vi "Update Call Chain.vi"(8 "error in (no error)":errorcluster, 11 "Data Cluster in":T1={"PeekVI Reference"=refnum, "SubPanel"=refnum, "Peek Stack Tree Ref"=refnum, "Open Button Ref"=refnum, "Top VI"=refnum, "Active VI"=refnum, "Stack"=[], "Last FP State"=enum."Standard"}) -> (0 "error out":errorcluster, 3 "Data Cluster out":T1={"PeekVI Reference"=refnum, "SubPanel"=refnum, "Peek Stack Tree Ref"=refnum, "Open Button Ref"=refnum, "Top VI"=refnum, "Active VI"=refnum, "Stack"=[], "Last FP State"=enum."Standard"})   [LabVIEW 2020, in "Peek Window.lvlib"]
uses:
  Peek Window.lvlib
  MHL Data Cluster.ctl
  VI Types/Standard VI Type/Standard VI Type.lvclass
  <vilib>/Utility/traverseref.llb/TRef TravTarget.ctl
  VI Types/Standard VI Type/Standard VI Type.lvclass/Standard VI Type.ctl
  VI Types/Standard VI Type/Read Full Qualified Name.vi
  <vilib>/Utility/traverseref.llb/VI Scripting - Traverse.lvlib
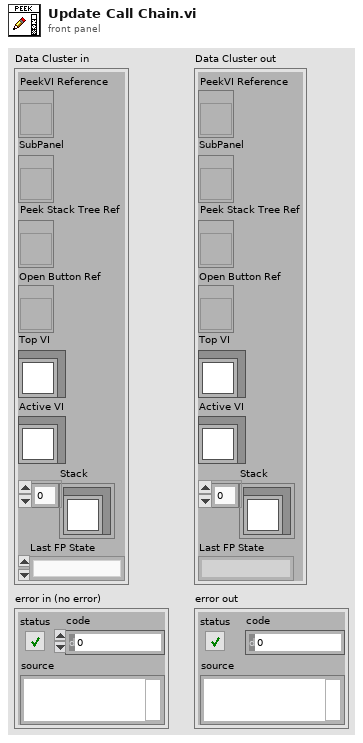
[diagram p1: front panel]
types:
  T1 = typedef "Peek Window.lvlib/MHL Data Cluster.ctl" = cluster{"PeekVI Reference":refnum<vi>, "SubPanel":refnum<vi>, "Peek Stack Tree Ref":refnum<vi>, "Open Button Ref":refnum<vi>, "Top VI":refnum<class "Standard VI Type.lvclass">, "Active VI":refnum<class "Standard VI Type.lvclass">, "Stack":refnum<class "Standard VI Type.lvclass">[], "Last FP State":enum32{"Invalid", "Standard", "Closed", "Hidden", "Minimized", "Maximized"}}
  T2 = typedef "TRef TravTarget.ctl" = enum16{"FP", "BD", "Other"}
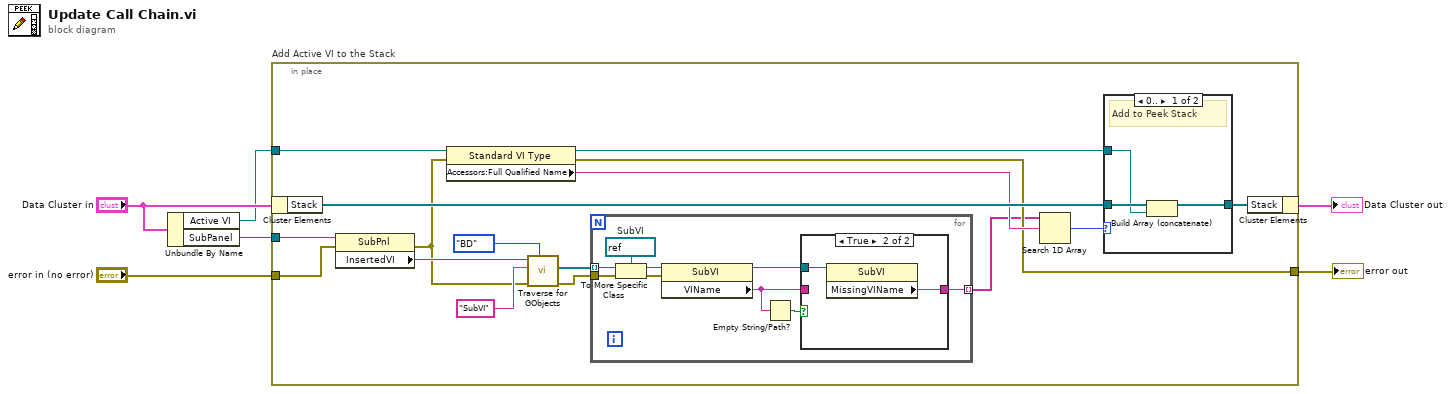
[diagram p0: block diagram]
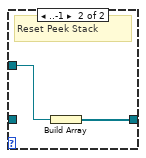
[diagram p3: hidden frame]
diagram:
  n1 = Unbundle By Name("Data Cluster in") -> ("Active VI"=w1:refnum<class "Standard VI Type.lvclass">, "SubPanel"=w6:refnum<vi>)
  n2 = in-place "Add Active VI to the Stack" {
    in-place-border: w6 -> [w22]
    in-place-border: w1 -> [w18]
    in-place-border: "error in (no error)" -> [w15]
    in-place-border: [w8] -> w4
    n3 = in-place-cluster #1("Data Cluster in") -> ("Stack"=w13:refnum<class "Standard VI Type.lvclass">[])
    n4 = property class="SubPnl"(reference=w22, error in=w15) -> (error out=w9:errorcluster, "InsertedVI"=w16:refnum<vi>)  [unwired: 1 out]
    n5 = property class="Standard VI Type"(reference=w18, error in=w9) -> (reference out=w11:refnum<class "Standard VI Type.lvclass">, error out=w8:errorcluster, "Accessors:Full Qualified Name"=w10:string)
    n6 = call <vilib>:"Traverse for GObjects.vi"("Traverse Target"=TRef_TravTarget."BD", "error in (no error)"=w9, "Class Name"="SubVI", "VI Refnum"=w16) -> ("error out"=w17:errorcluster, "References"=w19:refnum<vi>[])  [unwired: 4 in, 2 out]
    n7 = for {
      tunnel: w19 -> [w31] mode=indexing
      tunnel: w17 -> [w28]
      tunnel: [w23] -> w7 mode=indexing
      w30 = refnum<vi> refnum  # SubVI
      n8 = To More Specific Class(target class=w30, reference=w31, error in=w28) -> (specific class reference=w29:refnum<vi>, error out=w27:errorcluster)
      n9 = property class="SubVI"(reference=w29, error in=w27) -> (reference out=w26:refnum<vi>, "VIName"=w24:string)  [unwired: 1 out]
      n10 = Empty String/Path?(string/path=w24) -> (empty?=w25:bool)
      n11 = case shown="True" w25 {
        tunnel: w26 -> [_ w34]
        tunnel: w24 -> [w32 _]
        tunnel: [w32 w33] -> w23
        frame False {
        }
        frame True {
          n12 = property class="SubVI"(reference=w34) -> ("MissingVIName"=w33:string)  [unwired: 1 in, 2 out]
        }
      }
    }
    n13 = Search 1D Array(1D array=w7, element=w10) -> (index of element=w14:i32)  [unwired: 1 in]
    n14 = case shown="0.." w14 {
      tunnel: w11 -> [w36 w39]
      tunnel: [w35 w38] -> w12
      tunnel: w13 -> [w37 _]
      frame 0.. {
        # "Add to Peek Stack"
        n15 = Build Array (concatenate)(w37, w36) -> (w35:refnum<class "Standard VI Type.lvclass">[])
      }
      frame ..-1 {
        # "Reset Peek Stack"
        n16 = Build Array(w39) -> (w38:refnum<class "Standard VI Type.lvclass">[])
      }
    }
    n17 = in-place-cluster #1("Stack"=w12) -> (→"Data Cluster out":T1)
  }
  "error out" <- w4
